vi "Set All Controls Description.vi"(8 "Error In":errorcluster, 9 "Description":string, 11 "VI Ref":refnum<vi>) -> (0 "Error Out":errorcluster)   [LabVIEW 2021, in "Utilities.lvlib"]
uses:
  Utilities.lvlib
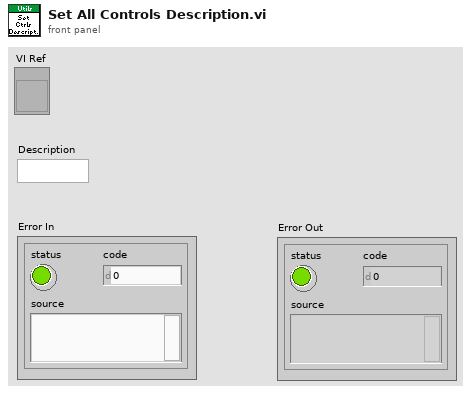
[diagram p1: front panel]
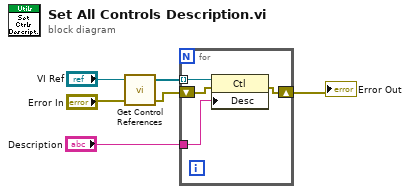
[diagram p0: block diagram]
diagram:
  n1 = call "Get Control References.vi"("error in"="Error In", "VI  Ref"="VI Ref") -> ("error out"=w3:errorcluster, "Controls[]"=w5:refnum<vi>[])  [unwired: 1 in, 1 out]
  n2 = for {
    tunnel: w5 -> [w10] mode=indexing
    shift-right: [w8] -> w2
    shift-left: w3 -> [w9]
    tunnel: "Description" -> [w7]
    n3 = property class="Ctl"(reference=w10, error in=w9, "Desc"=w7) -> (error out=w8:errorcluster)  [unwired: 1 out]
  }
  "Error Out" <- w2
